vi "Latihan 15 (Akar dan Kuadrat Polinomial).vi"() -> ()   [LabVIEW 2021]
uses:
  <vilib>/Analysis/polynomials.llb/Polynomial Roots (DBL).vi
  <vilib>/Analysis/polynomials.llb/Create Polynomial From Roots (CDB).vi
  <vilib>/Analysis/NI_AALPro.lvlib
panel:
  out "P(x) 2":dbl[](array[numeric]) format="%#.6g"
  out "Roots":cdb[](array[numeric])
  in  "P(x)":dbl[](array[numeric])
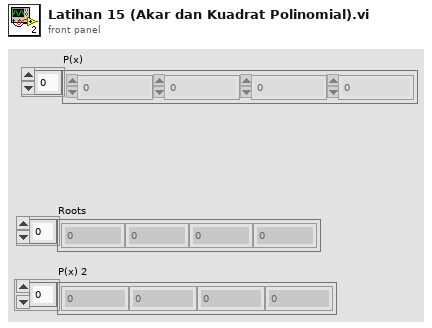
[diagram p1: front panel]
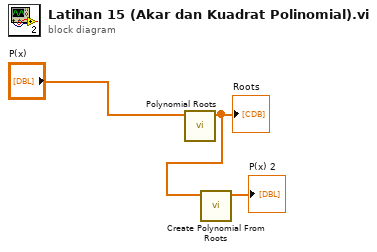
[diagram p0: block diagram]
diagram:
  n1 = call-poly <vilib>:"Polynomial Roots.vi"("P(x)"="P(x)") -> ("Roots"=w1:cdb[])  [unwired: 9 in, 1 out]
  "Roots" <- w1
  n2 = call-poly <vilib>:"Create Polynomial From Roots.vi"("Roots"=w1) -> ("P(x)"=→"P(x) 2":cdb[])  [unwired: 9 in, 1 out]
